vi "Create IWelcomeHandler.vi"(8 "error in (no error)":errorcluster, 11 "IWampMessage":refnum<class "IWampMessage.lvclass">) -> (0 "error out":errorcluster, 3 "IWelcomeHandler out":refnum<class "IWelcomeHandler.lvclass">)   [LabVIEW 2020, in "wamplv.lvlib"]
uses:
  wamplv.lvlib
  SerialisedMessages/JSONMessage/WampMessage JSON.lvclass
  SerialisedMessages/MsgPackMessage/WampMessage MsgPack.lvclass
  SerialisedMessages/IWampMessage/IWampMessage.lvclass
  IWelcomeHandler/IWelcomeHandler.lvclass
  WelcomeHandler MsgPack/WelcomeHandler MsgPack.lvclass
  WelcomeHandler JSON/WelcomeHandler JSON.lvclass
  C:/local/wamplv/Private/Requests/MessageReceivedHandlers/IJsonMessageHandler/IJsonMessageHandler.lvclass
  C:/local/wamplv/Private/Requests/MessageReceivedHandlers/IReceivedMessageHandler/IReceivedMessageHandler.lvclass
  C:/local/wamplv/Private/Requests/IInternalMessage/IInternalMessage.lvclass
  C:/local/wamplv/Private/Requests/MessageReceivedHandlers/Welcome/IWelcomeHandler/IWelcomeHandler.lvclass
  C:/local/wamplv/Private/Requests/MessageReceivedHandlers/WelcomeHandler JSON/WelcomeHandler JSON.lvclass
  C:/local/wamplv/Private/Requests/MessageReceivedHandlers/Welcome/WelcomeHandler MsgPack/WelcomeHandler MsgPack.lvclass
  C:/local/wamplv/Private/Requests/MessageReceivedHandlers/IMsgPackMessageHandler/IMsgPackMessageHandler.lvclass
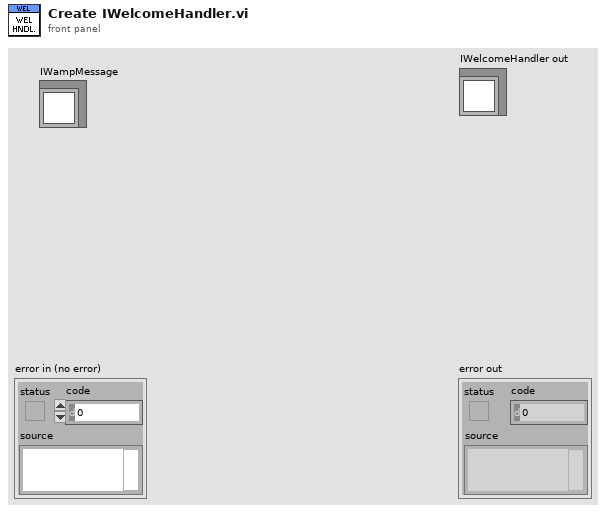
[diagram p1: front panel]
types:
  T1 = typedef "wamplv.lvlib/WAMP Client.lvclass/Serialisation.ctl" = enum16{"JSON", "MessagePack"}
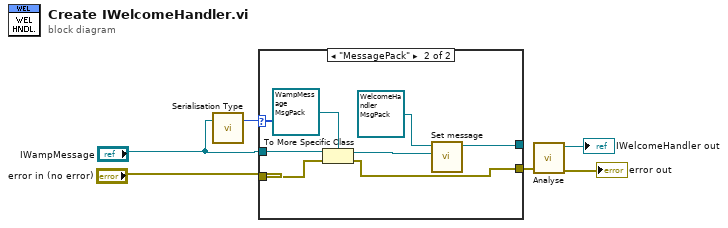
[diagram p0: block diagram]
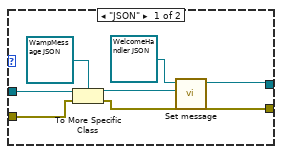
[diagram p2: hidden frame]
diagram:
  n1 = call-dynamic "Serialisation Type.vi"("IWampMessage in"="IWampMessage") -> ("Serialisation Type"=w6:T1)  [unwired: 2 in]
  n2 = case shown="\"MessagePack\"" w6 {
    tunnel: "IWampMessage" -> [w13 w20]
    tunnel: "error in (no error)" -> [w11 w19]
    tunnel: [w8 w15] -> w1
    tunnel: [w7 w14] -> _
    frame "JSON" {
      n3 = To More Specific Class(target class=refnum<class "WampMessage JSON.lvclass"> refnum ("wamplv.lvlib:JSONMessage.lvclass"), reference=w13, error in=w11) -> (specific class reference=w9:refnum<class "WampMessage JSON.lvclass">, error out=w8:errorcluster)
      n4 = call-dynamic "Set message.vi"("WampMessage JSON"=w9, "IMsgPackMessageHandler in"=refnum<class "WelcomeHandler JSON.lvclass"> refnum ("wamplv.lvlib:WelcomeHandler JSON.lvclass")) -> ("IMsgPackMessageHandler out"=w7:refnum<class "WelcomeHandler JSON.lvclass">)  [unwired: 9 in]
    }
    frame "MessagePack" {
      n5 = To More Specific Class(target class=refnum<class "WampMessage MsgPack.lvclass"> refnum ("wamplv.lvlib:MsgPackMessage.lvclass"), reference=w20, error in=w19) -> (specific class reference=w16:refnum<class "WampMessage MsgPack.lvclass">, error out=w15:errorcluster)
      n6 = call-dynamic "Set message.vi"("wamplv.lvlib:WampMessage MsgPack.lvclass"=w16, "WelcomeHandler MsgPack in"=refnum<class "WelcomeHandler MsgPack.lvclass"> refnum ("wamplv.lvlib:WelcomeHandler MsgPack.lvclass")) -> ("WelcomeHandler MsgPack out"=w14:refnum<class "WelcomeHandler MsgPack.lvclass">)  [unwired: 9 in]
    }
  }
  n7 = call-dynamic "Analyse.vi"("error in (no error)"=w1) -> ("error out"=→"error out":errorcluster, "IWelcomeHandler out"=→"IWelcomeHandler out":refnum<class "IWelcomeHandler.lvclass">)  [unwired: 9 in]
